vi "SAC-Apply Window.vi"(0 "Array in":cdb[](array[numeric]), 7 "Window":T1, 9 "Fs (Hz)":dbl) -> (4 "Array out":cdb[](array[numeric]))   [LabVIEW 2020]
uses:
  HRTF VIs/Typedefs/HRTF-Window.ctl
  HRTF VIs/Typedefs/HRTF-Window Type.ctl
  <vilib>/Analysis/2dsp.llb/Inverse Real FFT.vi
  <vilib>/Analysis/4window.llb/Hanning Window (DBL).vi
  <vilib>/Analysis/2dsp.llb/Complex FFT.vi
  <vilib>/Analysis/baseanly.llb/Mean.vi
  <vilib>/Analysis/baseanly.llb/Mean (DBL).vi
  <vilib>/Analysis/4window.llb/AllCosWindow (DBL).vi
  <vilib>/Analysis/NI_AALPro.lvlib
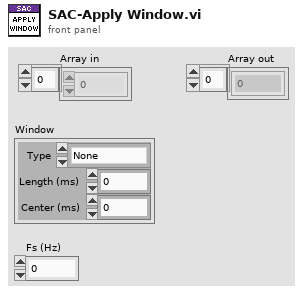
[diagram p1: front panel]
types:
  T1 = typedef "HRTF-Window.ctl" = cluster{"Type":T2, "Length (ms)":dbl, "Center (ms)":dbl}
  T2 = typedef "HRTF-Window Type.ctl" = enum16{"None", "Rectangle", "Hanning"}
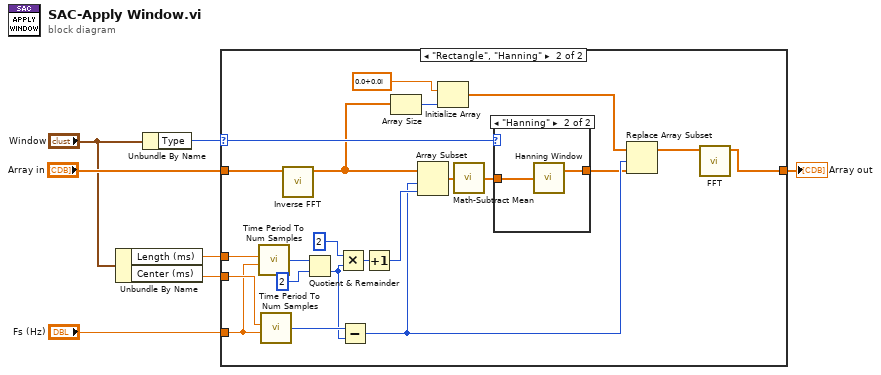
[diagram p0: block diagram]
diagram:
  n1 = Unbundle By Name("Window") -> ("Length (ms)"=w5:dbl, "Center (ms)"=w4:dbl)
  n2 = Unbundle By Name("Window") -> ("Type"=w2:T2)
  n3 = case shown="\"Rectangle\", \"Hanning\"" w2 {
    selector: w2 -> [_ w17]
    tunnel: "Array in" -> [w8 w24]
    tunnel: [w8 w9] -> w6
    tunnel: w5 -> [_ w30]
    tunnel: w4 -> [_ w29]
    tunnel: "Fs (Hz)" -> [_ w28]
    frame "None", Default {
    }
    frame "Rectangle", "Hanning" {
      n4 = call "Time Period To Num Samples.vi"("Duration (ms)"=w30, "Sampling rate (Hz)"=w28) -> ("Samples"=w26:i32)  [unwired: 5 in]
      n5 = call "Time Period To Num Samples.vi"("Duration (ms)"=w29, "Sampling rate (Hz)"=w28) -> ("Samples"=w25:i32)  [unwired: 5 in]
      n6 = call-poly <vilib>:"Inverse FFT.vi"("FFT {X}"=w24) -> ("X"=w16:dbl[])  [unwired: 9 in, 1 out]
      n7 = Quotient & Remainder(x=w26, y=2) -> (floor(x/y)=w23:i32)  [unwired: 1 out]
      n8 = Multiply(x=2, y=w23) -> (x*y=w21:i32)
      n9 = Subtract(x=w25, y=w23) -> (x-y=w12:i32)
      n10 = Increment(x=w21) -> (x+1=w18:i32)
      n11 = Array Size(array=w16) -> (size(s)=w15:i32)
      n12 = Array Subset(array=w16, index=w12, length=w18) -> (w20:dbl[])
      n13 = Initialize Array(cdb 0.0+0.0i, w15) -> (w13:cdb[])
      n14 = call "Math-Subtract Mean.vi"("Y"=w20) -> ("Y - mean(Y)"=w19:dbl[])  [unwired: 4 in]
      n15 = case shown="\"Hanning\"" w17 {
        tunnel: [w31 w33] -> w11
        tunnel: w19 -> [w31 w32]
        frame "None", Default {
        }
        frame "Hanning" {
          n16 = call-poly <vilib>:"Hanning Window.vi"("X"=w32) -> ("Windowed X"=w33:dbl[])  [unwired: 1 out]
        }
      }
      n17 = Replace Array Subset(array=w13, new element=w11, index=w12) -> (w10:cdb[])
      n18 = call-poly <vilib>:"FFT.vi"("X"=w10) -> ("FFT {X}"=w9:cdb[])  [unwired: 9 in, 1 out]
    }
  }
  "Array out" <- w6
